vi "output.vi"() -> ()   [LabVIEW 2021]
doc: "I. Description:\nThis example demonstrates how to output a single Voltage Update (Sample) to an Analog Output Channel.\n\nII. Instructions for Running:\n1. Select the Physical Channel to correspond to where your signal is output on the DAQ device.\n2. Enter the Minimum and Maximum Voltage Ranges\nNote: Use the Acq One Sample example to verify you are generating the correct output on the DAQ device\n\nIII. Block Diagram Steps:\n1. Create an Analog Output Voltage Channel\n2. Use the Write VI to Output 1 Sample to 1 Channel on the Data\nAcquisition Card. \n3. Call the Clear Task VI to clear the Task.\n4. Use the popup dialog box to display an error if any. \n\nIV. I/O Connections Overview:\nMake sure your signal output terminal matches the Physical Channel I/O Control. For further connection information, refer to your hardware reference manual."
uses:
  <vilib>/userdefined/High Color/nirio_resource_hc.ctl
  <vilib>/FPGAPlugInAG/PCIe-7857/niLvFpga_Open_PCIe-7857.vi
  <vilib>/rvi/interface/common/dynamic/niFpgaDynamicAddResources.vi
  <vilib>/Utility/error.llb/Error Cluster From Error Code.vi
  <vilib>/rvi/errors/niLvFpgaAdjustHostInterfaceError.vi
  <vilib>/FPGAPlugInAG/Dynamic/niLvFpga_Close_Dynamic.vi
  <vilib>/rvi/interface/nirviOpenFPGA/nirviOpenFPGA.xnode
  FPGA Bitfiles/lvfpga_FPGATarget_AO_PspK-PiI6Y0.lvbitx
  output_FPGA.vi
  <vilib>/rvi/interface/nirviReadWriteControl/nirviReadWriteControl.xnode
  <vilib>/rvi/interface/nirviCloseFPGA/nirviCloseFPGA.xnode
  NiFpgaLv.dll
  <vilib>/rvi/interface/Simulation/niFpgaSimulationCallBeginRW.vi
panel:
  in  "Tab Control":enum32{"Page 1", "Page 2"}(tab)
  in  "Data to Write":bool[](array[boolean])
  in  "开始循环":bool
  in  "停止循环":bool
  in  "保存数字控件":bool
  in  "读取数字控件":bool
  out "number":u32
  in  "stop":bool
  in  "AO Channels":dbl[](array[slide]) scale=-10.0..9.995 scale format="%.1f"
  in  "RIO Resource Name":T1="RIO0" caption="RIO Device"
  in  "Sample Clock Rate":dbl=200.0 format="%0.2f"
  out "16bit integer":i16[](array[numeric])
  # "Channel Parameters"
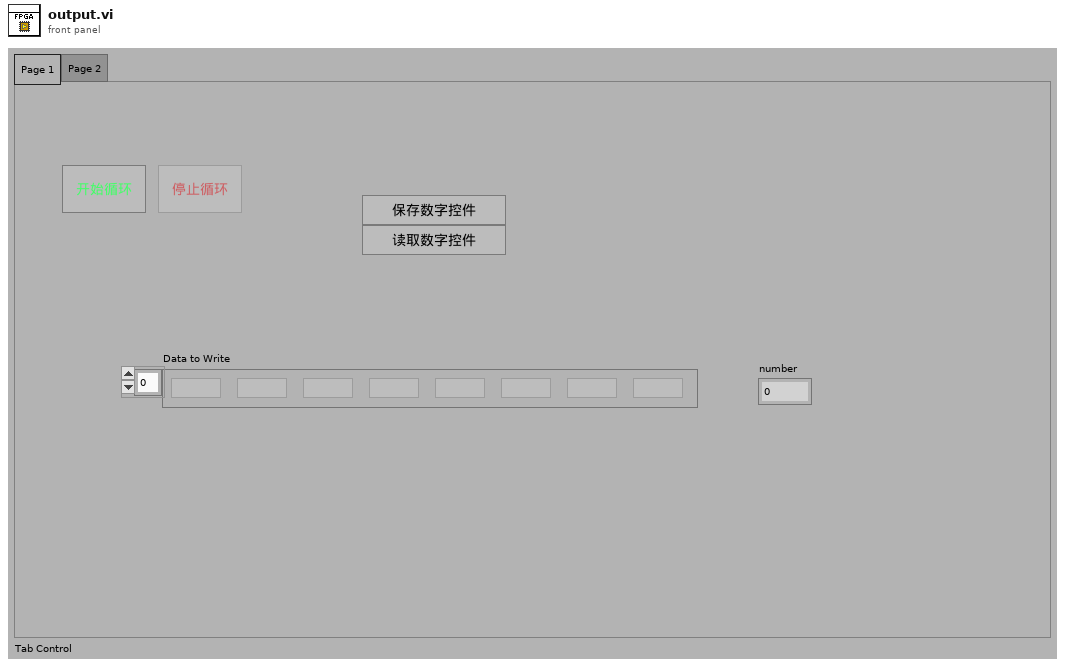
[diagram p1: front panel]
types:
  T1 = typedef "nirio_resource_hc.ctl" = tag
  T2 = enum8{"Enabled", "Disabled", "Disabled and Grayed Out"}
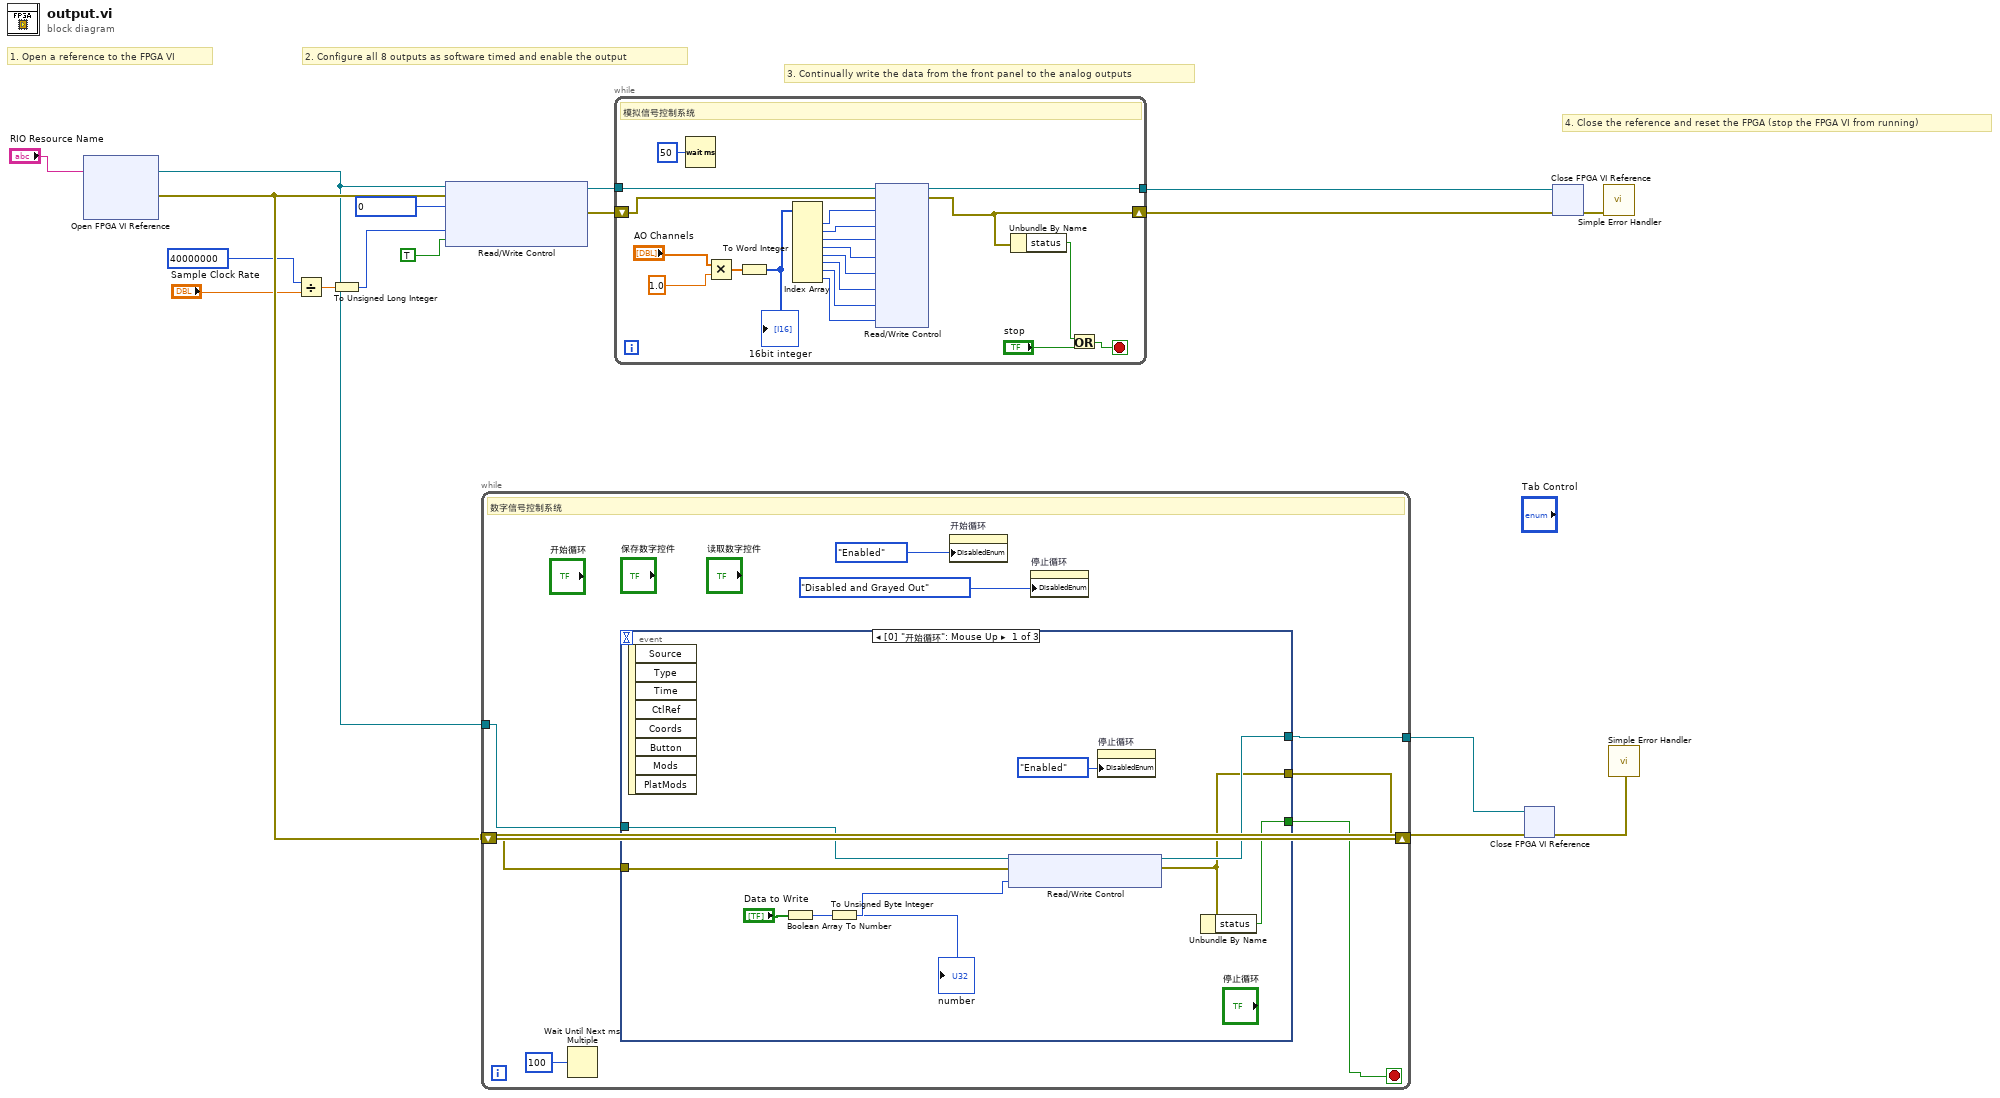
[diagram p0: block diagram]
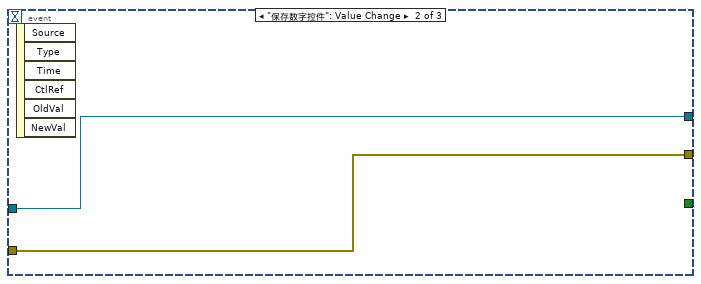
[diagram p2: hidden frame]
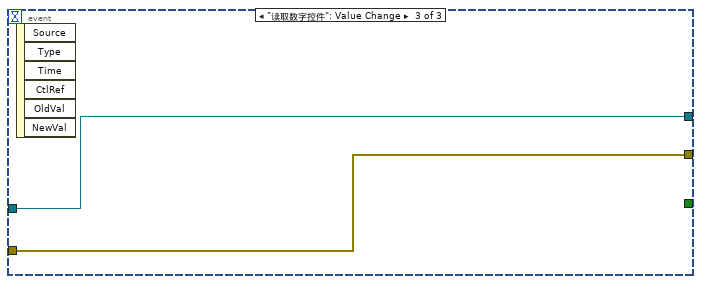
[diagram p3: hidden frame]
diagram:
  # "4. Close the reference and reset the FPGA (stop the FPGA VI from running)"
  # "3. Continually write the data from the front panel to the analog outputs"
  # "2. Configure all 8 outputs as software timed and enable the output"
  # "1. Open a reference to the FPGA VI"
  n1 = xnode ("Open FPGA VI Reference")("resource name"="RIO Resource Name") -> ("FPGA VI Reference Out"=w5:refnum<k20>, "error out"=w6:errorcluster)  [unwired: 1 in]
  n2 = Divide(x=u32 40000000, y="Sample Clock Rate") -> (x/y=w3:dbl)
  n3 = To Unsigned Long Integer(number=w3) -> (unsigned 32bit integer=w1:u32)
  n4 = xnode "Read/Write Control"("FPGA VI Reference In"=w5, "error in"=w6, "AO Buffer Enable"=u8 0, "AO Loop Timer(Ticks)"=w1, "AO Enable"=TRUE) -> ("FPGA VI Reference Out"=w14:refnum<k20>, "error out"=w13:errorcluster)
  n5 = while {
    tunnel: w5 -> [w19]
    tunnel: [w21] -> w12
    shift-right: [w20] -> w11
    shift-left: w6 -> [w22]
    stop <- w18 stop-if-true
    # "数字信号控制系统"
    n6 = Wait Until Next ms Multiple(millisecond multiple=u32 100 ("milliseconds to wait")) -> ()  [unwired: 1 out]
    n7 = event shown="[0] \"开始循环\": Mouse Up" {
      selector: _ -> [_ _ _]
      dyn-events: _ -> [_ _ _]
      timeout: _ -> [_ _ _]
      tunnel: w19 -> [w30 w36 w38]
      tunnel: w22 -> [w29 w35 w37]
      tunnel: [w28 _ _] -> w18
      tunnel: [w27 w36 w38] -> w21
      tunnel: [w26 w35 w37] -> w20
      event "开始循环": Mouse Up {
        n8 = event-data() -> ()  [unwired: 1 in, 8 out]
        n9 = Boolean Array To Number(Boolean array="Data to Write") -> (number=w31:u32)
        "number" <- w31
        n10 = To Unsigned Byte Integer(number=w31) -> (unsigned 8bit integer=w32:u8)
        n11 = xnode "Read/Write Control"("FPGA VI Reference In"=w30, "error in"=w29, "Connector 2 DIO Port 0"=w32) -> ("FPGA VI Reference Out"=w27:refnum<k20>, "error out"=w26:errorcluster)
        n12 = property on="停止循环" class="Bool"("DisabledEnum"=T2."Enabled" ("Disabled")) -> ()  [unwired: 2 in, 2 out]
        n13 = Unbundle By Name(w26) -> ("status"=w28:bool)
      }
      event "保存数字控件": Value Change {
        n14 = event-data() -> ()  [unwired: 1 in, 6 out]
      }
      event "读取数字控件": Value Change {
        n15 = event-data() -> ()  [unwired: 1 in, 6 out]
      }
    }
    n16 = property on="开始循环" class="Bool"("DisabledEnum"=T2."Enabled" ("Disabled")) -> ()  [unwired: 2 in, 2 out]
    n17 = property on="停止循环" class="Bool"("DisabledEnum"=T2."Disabled and Grayed Out" ("Disabled")) -> ()  [unwired: 2 in, 2 out]
  }
  n18 = while {
    tunnel: w14 -> [w58]
    shift-right: [w48] -> w16
    shift-left: w13 -> [w57]
    tunnel: [w49] -> w17
    stop <- w50 stop-if-true
    # "模拟信号控制系统"
    n19 = Wait (ms)(milliseconds to wait=u32 50) -> ()  [unwired: 1 out]
    n20 = Multiply(x="AO Channels", y=1.0) -> (x*y=w55:dbl[])
    n21 = To Word Integer(number=w55) -> (16bit integer=w54:i16[])
    "16bit integer" <- w54
    n22 = Index Array(array=w54) -> (element #1=w46:i16, element #2=w45:i16, element #3=w44:i16, element #4=w43:i16, element #5=w42:i16, element #6=w41:i16, element #7=w40:i16, element #8=w39:i16)  [unwired: 8 in]
    n23 = xnode "Read/Write Control"("FPGA VI Reference In"=w58, "error in"=w57, "AO 0"=w46, "AO 1"=w45, "AO 2"=w44, "AO 3"=w43, "AO 4"=w42, "AO 5"=w41, "AO 6"=w40, "AO 7"=w39) -> ("FPGA VI Reference Out"=w49:refnum<k20>, "error out"=w48:errorcluster)
    n24 = Unbundle By Name(w48) -> ("status"=w51:bool)
    n25 = Or(x=w51, y="stop") -> (x .or. y?=w50:bool)
  }
  n26 = xnode "Close FPGA VI Reference"("FPGA VI Reference In"=w12, "error in"=w11) -> ("error out"=w10:errorcluster)
  n27 = xnode "Close FPGA VI Reference"("FPGA VI Reference In"=w17, "error in"=w16) -> ("error out"=w15:errorcluster)
  n28 = call <vilib>:"Simple Error Handler.vi"("error in (no error)"=w15) -> ()  [unwired: 4 in, 5 out]
  n29 = call <vilib>:"Simple Error Handler.vi"("error in (no error)"=w10) -> ()  [unwired: 4 in, 5 out]
